vi "spec_set_cupconfig.vi"(8 "error in (no error)":errorcluster, 9 "supcub config name":string, 10 "cup config name":string, 11 "instrument in":refnum<class "instrument.lvclass">) -> (0 "error out":errorcluster, 2 "value out":string, 3 "instrument out":refnum<class "instrument.lvclass">)   [LabVIEW 2018, in "instrument.lvclass"]
doc: "set the cup and subcup configuration of the instrument\n\nmainly for qtegra"
uses:
  instrument.lvclass
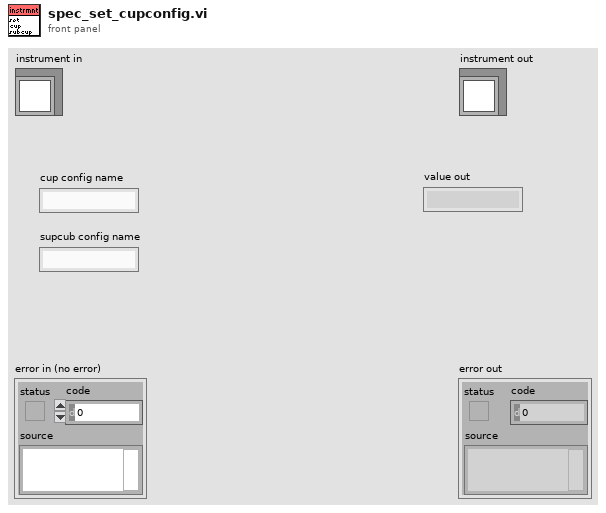
[diagram p1: front panel]
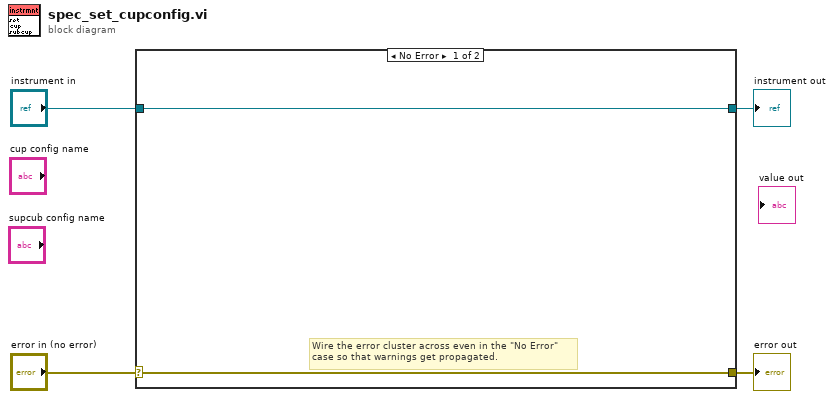
[diagram p0: block diagram]
diagram:
  n1 = case shown="No Error" "error in (no error)" {
    selector: "error in (no error)" -> [w5 w8]
    tunnel: [w5 w8] -> w3
    tunnel: [w6 w7] -> w1
    tunnel: "instrument in" -> [w6 w7]
    frame No Error {
      # "Wire the error cluster across even in the \"No Error\"\ncase so that warnings get propagated."
    }
    frame Error {
    }
  }
  "error out" <- w3
  "instrument out" <- w1
